vi "water flow PID.vi"(5 "Time":dbl format="%.2f", 6 "sensor value":dbl, 7 "Set Points":dbl[](array[numeric])) -> (1 "required number of setpoints":u8, 2 "Set Point names":string[](array[string]), 3 "fraction on":dbl)   [LabVIEW 2010]
uses:
  <userlib>/Process Controller 3.0/control code old/water flow PID.vi/PID (DBL).vi
panel:
  in  "PID gains":T1={"proportional gain (Kc)"=1.0, "integral time (Ti, min)"=0.0, "derivative time (Td, min)"=0.0} {"derivative time (Td, min)" format="%.3f"; "integral time (Ti, min)" format="%.3f"; "proportional gain (Kc)" format="%.3f"}
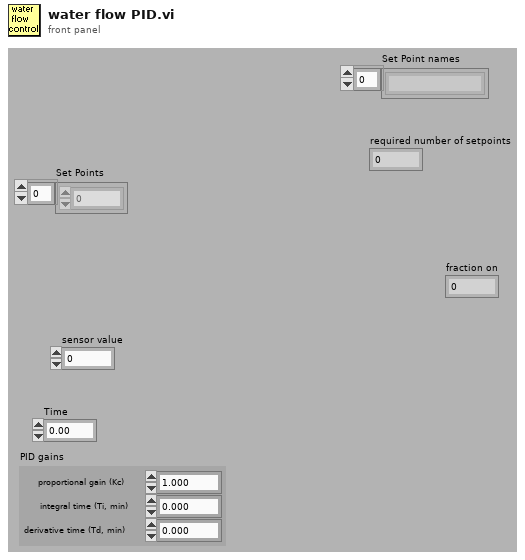
[diagram p1: front panel]
types:
  T1 = cluster{"proportional gain (Kc)":dbl, "integral time (Ti, min)":dbl, "derivative time (Td, min)":dbl}
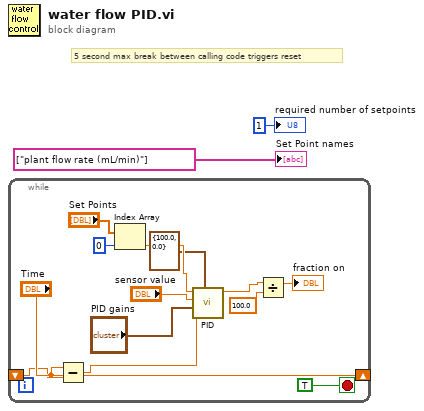
[diagram p0: block diagram]
diagram:
  # "5 second max break between calling code triggers reset"
  n1 = while {
    shift-right: ["Time"] -> _
    shift-left: _ -> [w10]
    stop <- TRUE stop-if-true
    n2 = Subtract(x="Time", y=w10) -> (x-y=w9:dbl)
    n3 = Index Array(array="Set Points", index=0) -> (element=w12:dbl)
    n4 = call-poly "PID.vi"("output range"=cluster{"output high":dbl, "output low":dbl} {"output high"=100.0, "output low"=0.0}, "dt (s)"=w9, "PID gains"="PID gains", "process variable"="sensor value", "setpoint"=w12) -> ("output"=w6:dbl)  [unwired: 5 in, 1 out]
    n5 = Divide(x=w6, y=100.0) -> (x/y=→"fraction on":dbl)
  }
  "Set Point names" <- string[] ["plant flow rate (mL/min)"] ("Set Point names")
  "required number of setpoints" <- u8 1 ("required number of setpoints")
